vi "mainVI.vi"() -> ()   [LabVIEW 2017]
panel:
  in  "ID":string
  in  "GET ID Button":bool
  in  "stop":bool
  in  "VISA resource name":refnum<visa-resource-name>
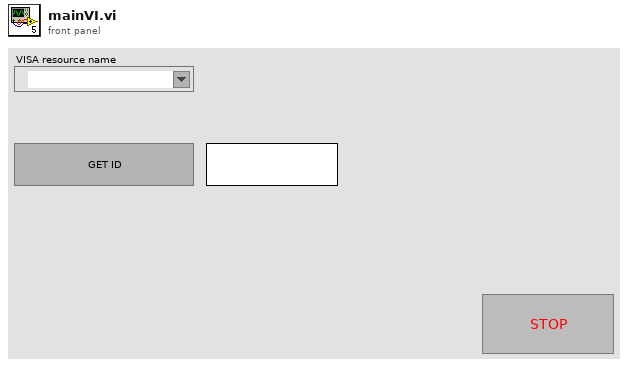
[diagram p1: front panel]
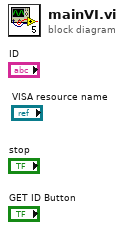
[diagram p0: block diagram]
diagram:
